vi "Count Number of Measurements for a Part.vi"(10 "Part Name":string, 11 "AllPartInfoArray":T1) -> (3 "Number of Measurements":i32)   [LabVIEW 2019, in "DataLogger.lvclass"]
uses:
  DataLogger.lvclass
  Common/Controls/AllPartInfo.ctl
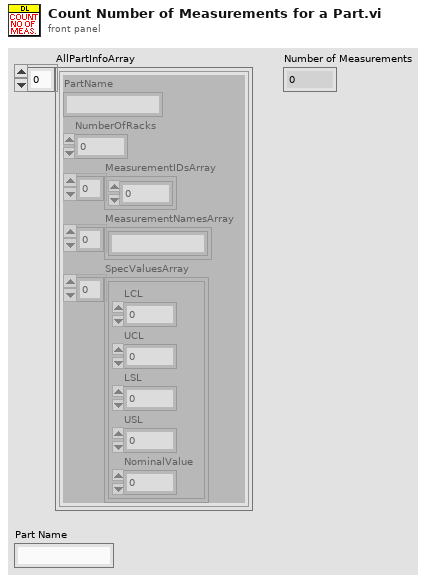
[diagram p1: front panel]
types:
  T1 = typedef "AllPartInfo.ctl" = cluster{"PartName":string, "NumberOfRacks":u8, "MeasurementIDsArray":u16[], "MeasurementNamesArray":string[], "SpecValuesArray":cluster{"LCL":dbl, "UCL":dbl, "LSL":dbl, "USL":dbl, "NominalValue":dbl}[]}[]
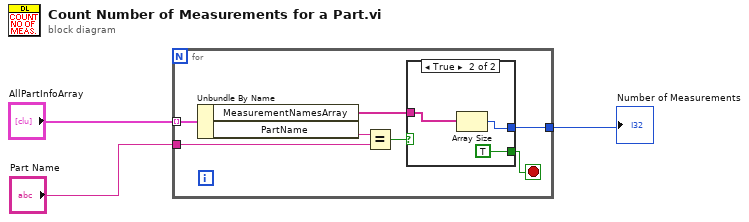
[diagram p0: block diagram]
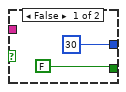
[diagram p2: hidden frame]
diagram:
  n1 = for {
    tunnel: "AllPartInfoArray" -> [w10] mode=indexing
    tunnel: "Part Name" -> [w8]
    tunnel: [w5] -> w1
    stop <- w4 stop-if-true
    n2 = Unbundle By Name(w10) -> ("MeasurementNamesArray"=w6:string[], "PartName"=w9:string)
    n3 = Equal?(x=w9, y=w8) -> (x = y?=w7:bool)
    n4 = case shown="True" w7 {
      tunnel: w6 -> [_ w15]
      tunnel: [30 w14] -> w5
      tunnel: [FALSE TRUE] -> w4
      frame False {
      }
      frame True {
        n5 = Array Size(array=w15) -> (size(s)=w14:i32)
      }
    }
  }
  "Number of Measurements" <- w1
